vi "Check Multiple Computers Awake using Ping.vi"(11 "List of IPs":string[](array[string])) -> (0 "ping times [ms]":u32[](array[numeric]), 2 "Awake?":bool[](array[boolean]), 3 "List of IPs out":string[](array[string]))   [LabVIEW 2013]
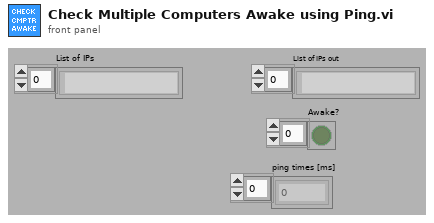
[diagram p1: front panel]
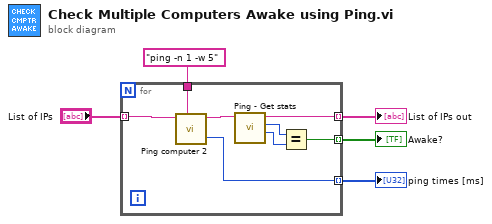
[diagram p0: block diagram]
diagram:
  n1 = for {
    tunnel: "List of IPs" -> [w13] mode=indexing
    tunnel: "ping -n 1 -w 5" ("Ping Command (ping -n 1 -w 5)") -> [w11]
    tunnel: [w10] -> w3 mode=indexing
    tunnel: [w9] -> w2 mode=indexing
    tunnel: [w6] -> w1 mode=indexing
    n2 = call "Ping computer 2.vi"("Ping Command (ping -n 1 -w 5)"=w11, "IP Address"=w13) -> ("Ping Output"=w12:string, "ping time [ms]"=w10:u32)  [unwired: 2 in, 6 out]
    n3 = call "Ping - Get stats.vi"("Ping Output"=w12) -> ("# of packets received"=w7:i32, "# of packets sent"=w8:i32, "IP Address"=w9:string)  [unwired: 8 out]
    n4 = Equal?(x=w8, y=w7) -> (x = y?=w6:bool)
  }
  "List of IPs out" <- w2
  "ping times [ms]" <- w3
  "Awake?" <- w1
